vi "CircleDataBuffer.vi"() -> ()   [LabVIEW 2011]
uses:
  <vilib>/Analysis/1siggen.llb/Ramp Pattern by Samples.vi
  <vilib>/Analysis/NI_AALBase.lvlib
  <vilib>/ptbypt/NI_PtbyPt.lvlib
panel:
  out "XY Graph":T1(graph)
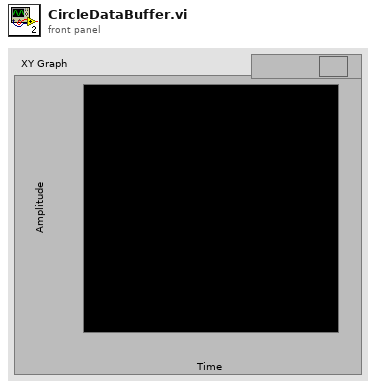
[diagram p1: front panel]
types:
  T1 = cluster{"Current Queue":dbl[], "Current Queue":dbl[]}
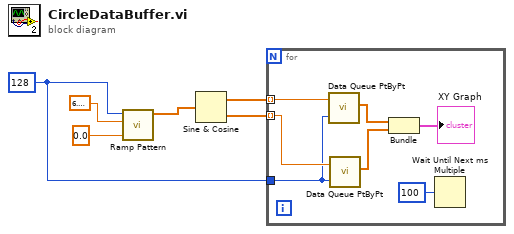
[diagram p0: block diagram]
diagram:
  w1 = 128 ("samples")
  n1 = call-poly <vilib>:"Ramp Pattern.vi"("start"=0.0, "end"=6.283185307179586, "samples"=w1) -> ("Ramp Pattern"=w4:dbl[])  [unwired: 7 in, 1 out]
  n2 = Sine & Cosine(0:w4) -> (1:w6:dbl[], 2:w5:dbl[])
  n3 = for {
    tunnel: w6 -> [w12] mode=indexing
    tunnel: w5 -> [w11] mode=indexing
    tunnel: w1 -> [w10]
    n4 = call <vilib>:"Data Queue PtByPt.vi"("input data point"=w12, "sample length"=w10) -> ("Current Queue"=w9:dbl[])  [unwired: 1 in, 4 out]
    n5 = call <vilib>:"Data Queue PtByPt.vi"("input data point"=w11, "sample length"=w10) -> ("Current Queue"=w8:dbl[])  [unwired: 1 in, 4 out]
    n6 = Bundle("Current Queue"=w9, "Current Queue"=w8) -> (→"XY Graph":T1)  [unwired: 1 in]
    n7 = Wait Until Next ms Multiple(millisecond multiple=u32 100) -> ()  [unwired: 1 out]
  }
